vi "BotSpeak_Wait.vi"(2 "Wait (sec)":dbl=1.0, 3 "Bot Settings":T1) -> (1 "Bot Settings":T1)   [LabVIEW 2012]
doc: "Causes VI to wait the specified number of seconds."
uses:
  <userlib>/BotSpeak/VIs/Direct/BotSpeak_Control.ctl
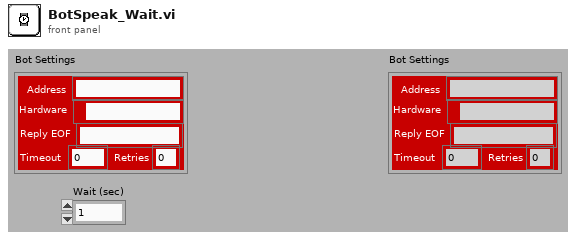
[diagram p1: front panel]
types:
  T1 = typedef "BotSpeak_Control.ctl" = cluster{"Address":string, "Reply EOF":string, "Hardware":path, "Retries":i8, "Timeout":i32}
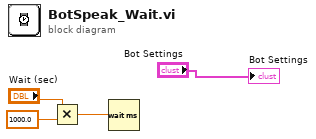
[diagram p0: block diagram]
diagram:
  n1 = Multiply(x="Wait (sec)", y=1000.0) -> (x*y=w1:dbl)
  n2 = Wait (ms)(milliseconds to wait=w1) -> ()  [unwired: 1 out]
  "Bot Settings" <- "Bot Settings"
